vi "Write json to AIParam one.vi"(8 "error in (no error)":errorcluster, 10 "JSON Data In":string, 11 "AI in":T1) -> (0 "error out":errorcluster, 3 "AI out":T1)   [LabVIEW 2019, in "Inputs.lvlib"]
doc: "sorting to fcode_full column\nfa_1 request returns fcode_full without ltree points GM1QN3_XQ01\nfa_3 request returns fcode_full with ltree points GM1.QN3_XQ01\n {\"GM1QN3_XQ01\":{\"instrument_gain\":10,\n \"input_register_min\":6554,\n \"input_register_max\":32767,\n \"input_pv_max\":2.5},\n \"GM1QN4_XQ01\":{\"instrument_gain\":10,\n \"input_register_min\":6554,\n \"input_register_max\":32767,\n \"input_pv_max\":4.99}\n}"
uses:
  Inputs.lvlib
  Ctl/AI.ctl
  Ctl/AI short.ctl
  Ctl/Parameter State.ctl
  Ctl/AIParamColumns.ctl
  <vilib>/JDP Science/JSONtext/Find Multiple Items.vi
  <vilib>/JDP Science/JSONtext/String Subset.vi
  <vilib>/JDP Science/JSONtext/support/Strip Quotes and Unescape.vi
  <vilib>/JDP Science/JSONtext/support/Unescape JSON string.vi
  <vilib>/JDP Science/JSONtext/Parsing/Parse Full Path or Item Name.vi
  <vilib>/JDP Science/JSONtext/Offset/Find Item Locations by Path.vi
  <vilib>/JDP Science/JSONtext/Get Array Elements.vi
  Userlib.lvlib
panel:
  # "Analog parameters"
  # "Description of analog parameters"
  # "Analog parameters"
  # "Description of analog parameters"
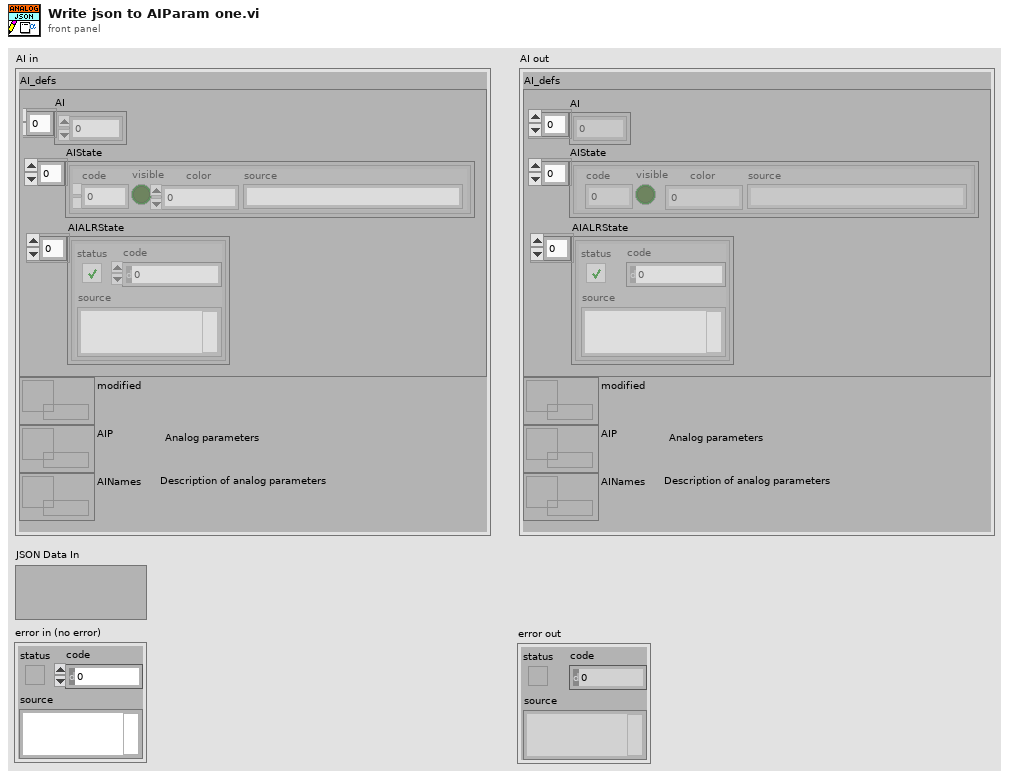
[diagram p1: front panel]
types:
  T1 = typedef "Inputs.lvlib/AI.ctl" = cluster{"AI_defs":T2, "modified":refnum<data-value>, "AIP":refnum<data-value>, "AINames":refnum<data-value>}
  T2 = typedef "Inputs.lvlib/AI short.ctl" = cluster{"AI":dbl[], "AIState":T3[], "AIALRState":errorcluster[]}
  T3 = typedef "Inputs.lvlib/Parameter State.ctl" = cluster{"code":i32, "visible":bool, "color":u32, "source":string}
  T4 = typedef "Inputs.lvlib/AIParamColumns.ctl" = enum16{"instrument_gain", "instrument_offset", "time_const", "instrument_min_offset", "instrument_range_min", "process_range_min", "process_low_acd", "process_low_alr", "process_high_alr", "process_high_acd", "process_range_max", "instrument_range_max", "instrument_max_offset", "d", "input_register_min", "input_register_max", "input_pv_min", "input_pv_max", "module_fcode_full", "control_channel_num", "ip_adress", "fcode", "fcodef", "fcode_full", "fname", "process_units"}
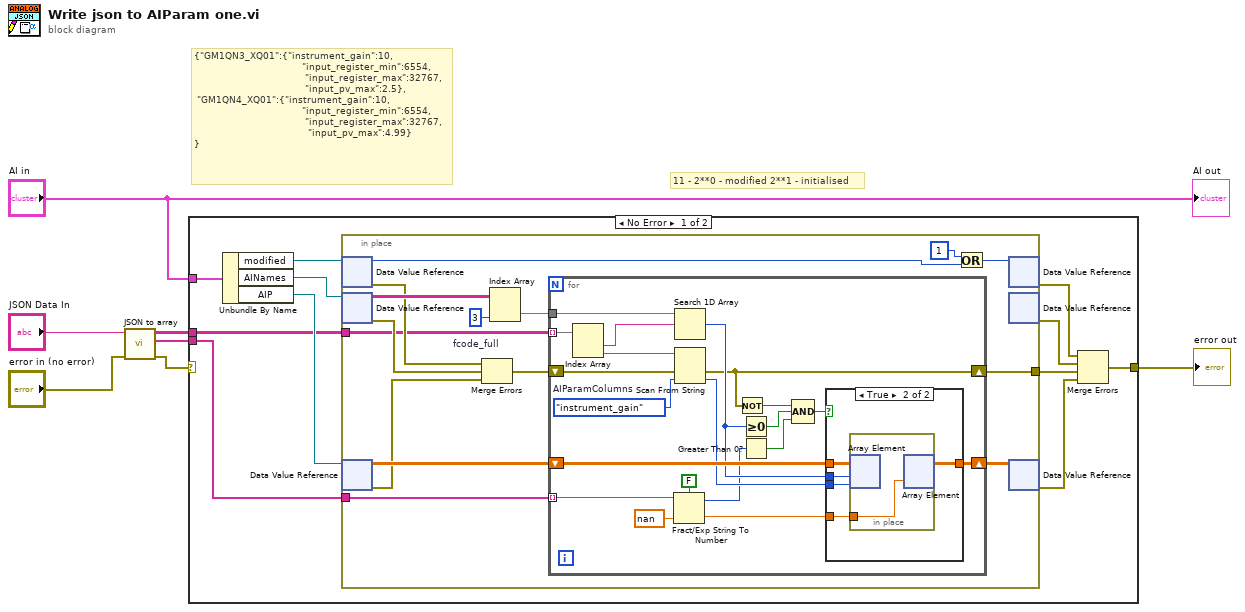
[diagram p0: block diagram]
diagram:
  # "{\"GM1QN3_XQ01\":{\"instrument_gain\":10,\n                                    \"input_register_min\":6554,\n                                     \"input_register_max\":32767,\n                                     \"input_pv_max\":2.5},\n \"GM1QN4_XQ01\":{\"instrument_gain\":10,\n                                    \"input_register_min\":6554,\n                                     \"input_register_max\":32767,\n                                      \"input_pv_max\":4.99}\n}"
  # "11 - 2**0 - modified 2**1 - initialised"
  n1 = call "JSON to array.vi"("error in (no error)"="error in (no error)", "JSON Data In"="JSON Data In") -> ("error out"=w1:errorcluster, "values"=w4:string[], "names"=w3:string[][])  [unwired: 7 in]
  n2 = case shown="No Error" w1 {
    selector: w1 -> [_ w61]
    tunnel: [w17 w61] -> w2
    tunnel: "AI in" -> [w18 _]
    tunnel: w4 -> [w15 _]
    tunnel: w3 -> [w10 _]
    frame No Error {
      n3 = Unbundle By Name(w18) -> ("modified"=w12:refnum<data-value>, "AINames"=w14:refnum<data-value>, "AIP"=w16:refnum<data-value>)
      n4 = in-place {
        in-place-border: w15 -> [w26]
        in-place-border: [w27] -> w8
        in-place-border: w10 -> [w20]
        w19 = 3  # fcode_full
        n5 = in-place-dvr #1(w12) -> (w24:u8, w22:errorcluster)
        n6 = in-place-dvr #2(w14) -> (w31:string[][], w29:errorcluster)
        n7 = in-place-dvr #3(w16) -> (w33:dbl[][], w28:errorcluster)
        n8 = Merge Errors(w22, w29, w28) -> (w21:errorcluster)
        n9 = Index Array(array=w31, index (col)=w19) -> (element=w30:string[])  [unwired: 1 in]
        n10 = for {
          tunnel: w30 -> [w51]
          tunnel: w26 -> [w49] mode=indexing
          shift-right: [w35] -> w27
          shift-left: w21 -> [w46]
          shift-right: [w52] -> w32
          shift-left: w33 -> [w53]
          tunnel: w20 -> [w45] mode=indexing
          w34 = AIParamColumns."instrument_gain"  # AIParamColumns
          n11 = Index Array(array=w45) -> (element #1=w44:string, element #2=w43:string)  [unwired: 2 in]
          n12 = Fract/Exp String To Number(use system decimal point (T)=FALSE, string=w49, default (0 dbl)=nan ("default (0 DBL)")) -> (offset past number=w40:i32, number=w48:dbl)  [unwired: 1 in]
          n13 = Search 1D Array(1D array=w51, element=w44) -> (index of element=w41:i32)  [unwired: 1 in]
          n14 = Scan From String(input string=w43, error in=w46, default 1=w34) -> (error out=w35:errorcluster, output 1=w50:T4)  [unwired: 2 in, 2 out]
          n15 = Not(x=w35) -> (.not. x?=w39:bool)
          n16 = Greater Or Equal To 0?(x=w41) -> (x >= 0?=w38:bool)
          n17 = Greater Than 0?(x=w40) -> (x > 0?=w37:bool)
          n18 = Compound Arithmetic op=AND(w39, w38, w37) -> (w36:bool)
          n19 = case shown="True" w36 {
            tunnel: w53 -> [w54 w59]
            tunnel: [w54 w58] -> w52
            tunnel: w50 -> [_ w57]
            tunnel: w48 -> [_ w56]
            tunnel: w41 -> [_ w55]
            frame False {
            }
            frame True {
              n20 = in-place {
                in-place-border: w56 -> [w60]
                n21 = in-place-array #4(w59, w55, w57) -> ()  [unwired: 1 out]
                n22 = in-place-array #4(w60) -> (w58:dbl[][])  [unwired: 2 out]
              }
            }
          }
        }
        n23 = Or(x=u8 1 ("data value"), y=w24) -> (x .or. y?=w23:u8)
        n24 = in-place-dvr #1(w23) -> (w11:errorcluster)  [unwired: 1 out]
        n25 = in-place-dvr #2() -> (w13:errorcluster)  [unwired: 1 in, 1 out]
        n26 = in-place-dvr #3(w32) -> (w9:errorcluster)  [unwired: 1 out]
      }
      n27 = Merge Errors(w11, w13, w8, w9) -> (w17:errorcluster)
    }
    frame Error {
    }
  }
  "error out" <- w2
  "AI out" <- "AI in"
